vi "frontPanel.vi"() -> ()   [LabVIEW 2020]
uses:
  C:/Users/DESKTOP-TLO0G68A/Desktop/instrumentationLV/Thorlabs.MotionControl.Controls.dll
  Thorlabs.MotionControl.Controls.dll
  C:/Users/DESKTOP-TLO0G68A/Desktop/instrumentationLV/ThorLabs.MotionControl.KCube.DCServoCLI.dll
  ThorLabs.MotionControl.KCube.DCServoCLI.dll
panel:
  in  "KCubeDCServoControl 1":refnum<k24>(container)
  in  "?":bool
  in  "?":bool
  in  "?":bool
  in  "Direction 2":i32(ring)=1 items=["Forward"=1, "Backward"=2]
  in  "Step Size 2":dbl
  in  "KCubeDCServoControl 2":refnum<k24>(container)
  in  "?":bool
  in  "?":bool
  in  "?":bool
  in  "Direction":i32(ring)=1 items=["Forward"=1, "Backward"=2]
  in  "Step Size":dbl
  in  "x steps":dbl
  in  "NPLC":dbl
  in  "# of pts":dbl
  in  "velocity":dbl
  in  "ending voltage":dbl
  in  "starting voltage":dbl
  in  "Oscilloscope VISA addr":refnum<visa-resource-name>
  in  "Keithley VISA addr":refnum<visa-resource-name>
  in  "acceleration":dbl
  in  "step size":dbl=0.025
  in  "y steps":dbl
  in  "Starting y":dbl
  in  "Starting x":dbl
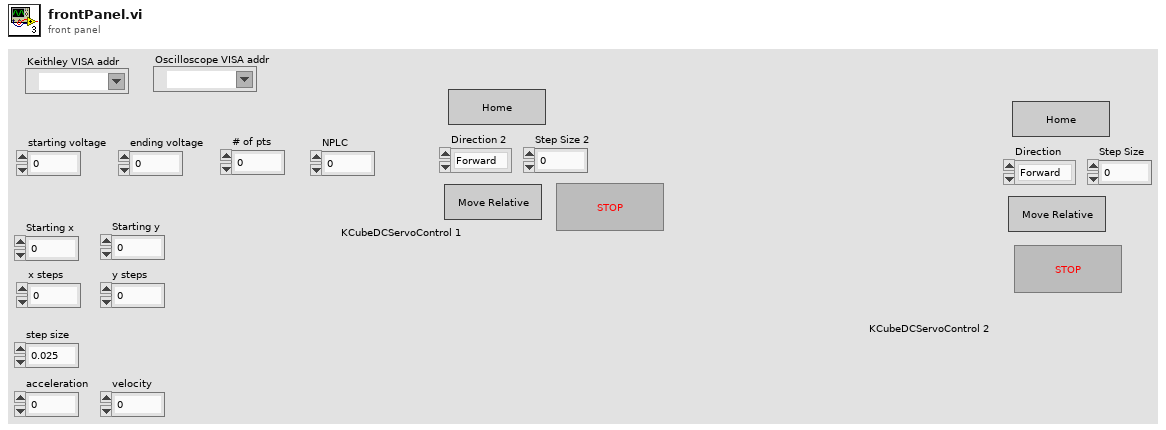
[diagram p1: front panel]
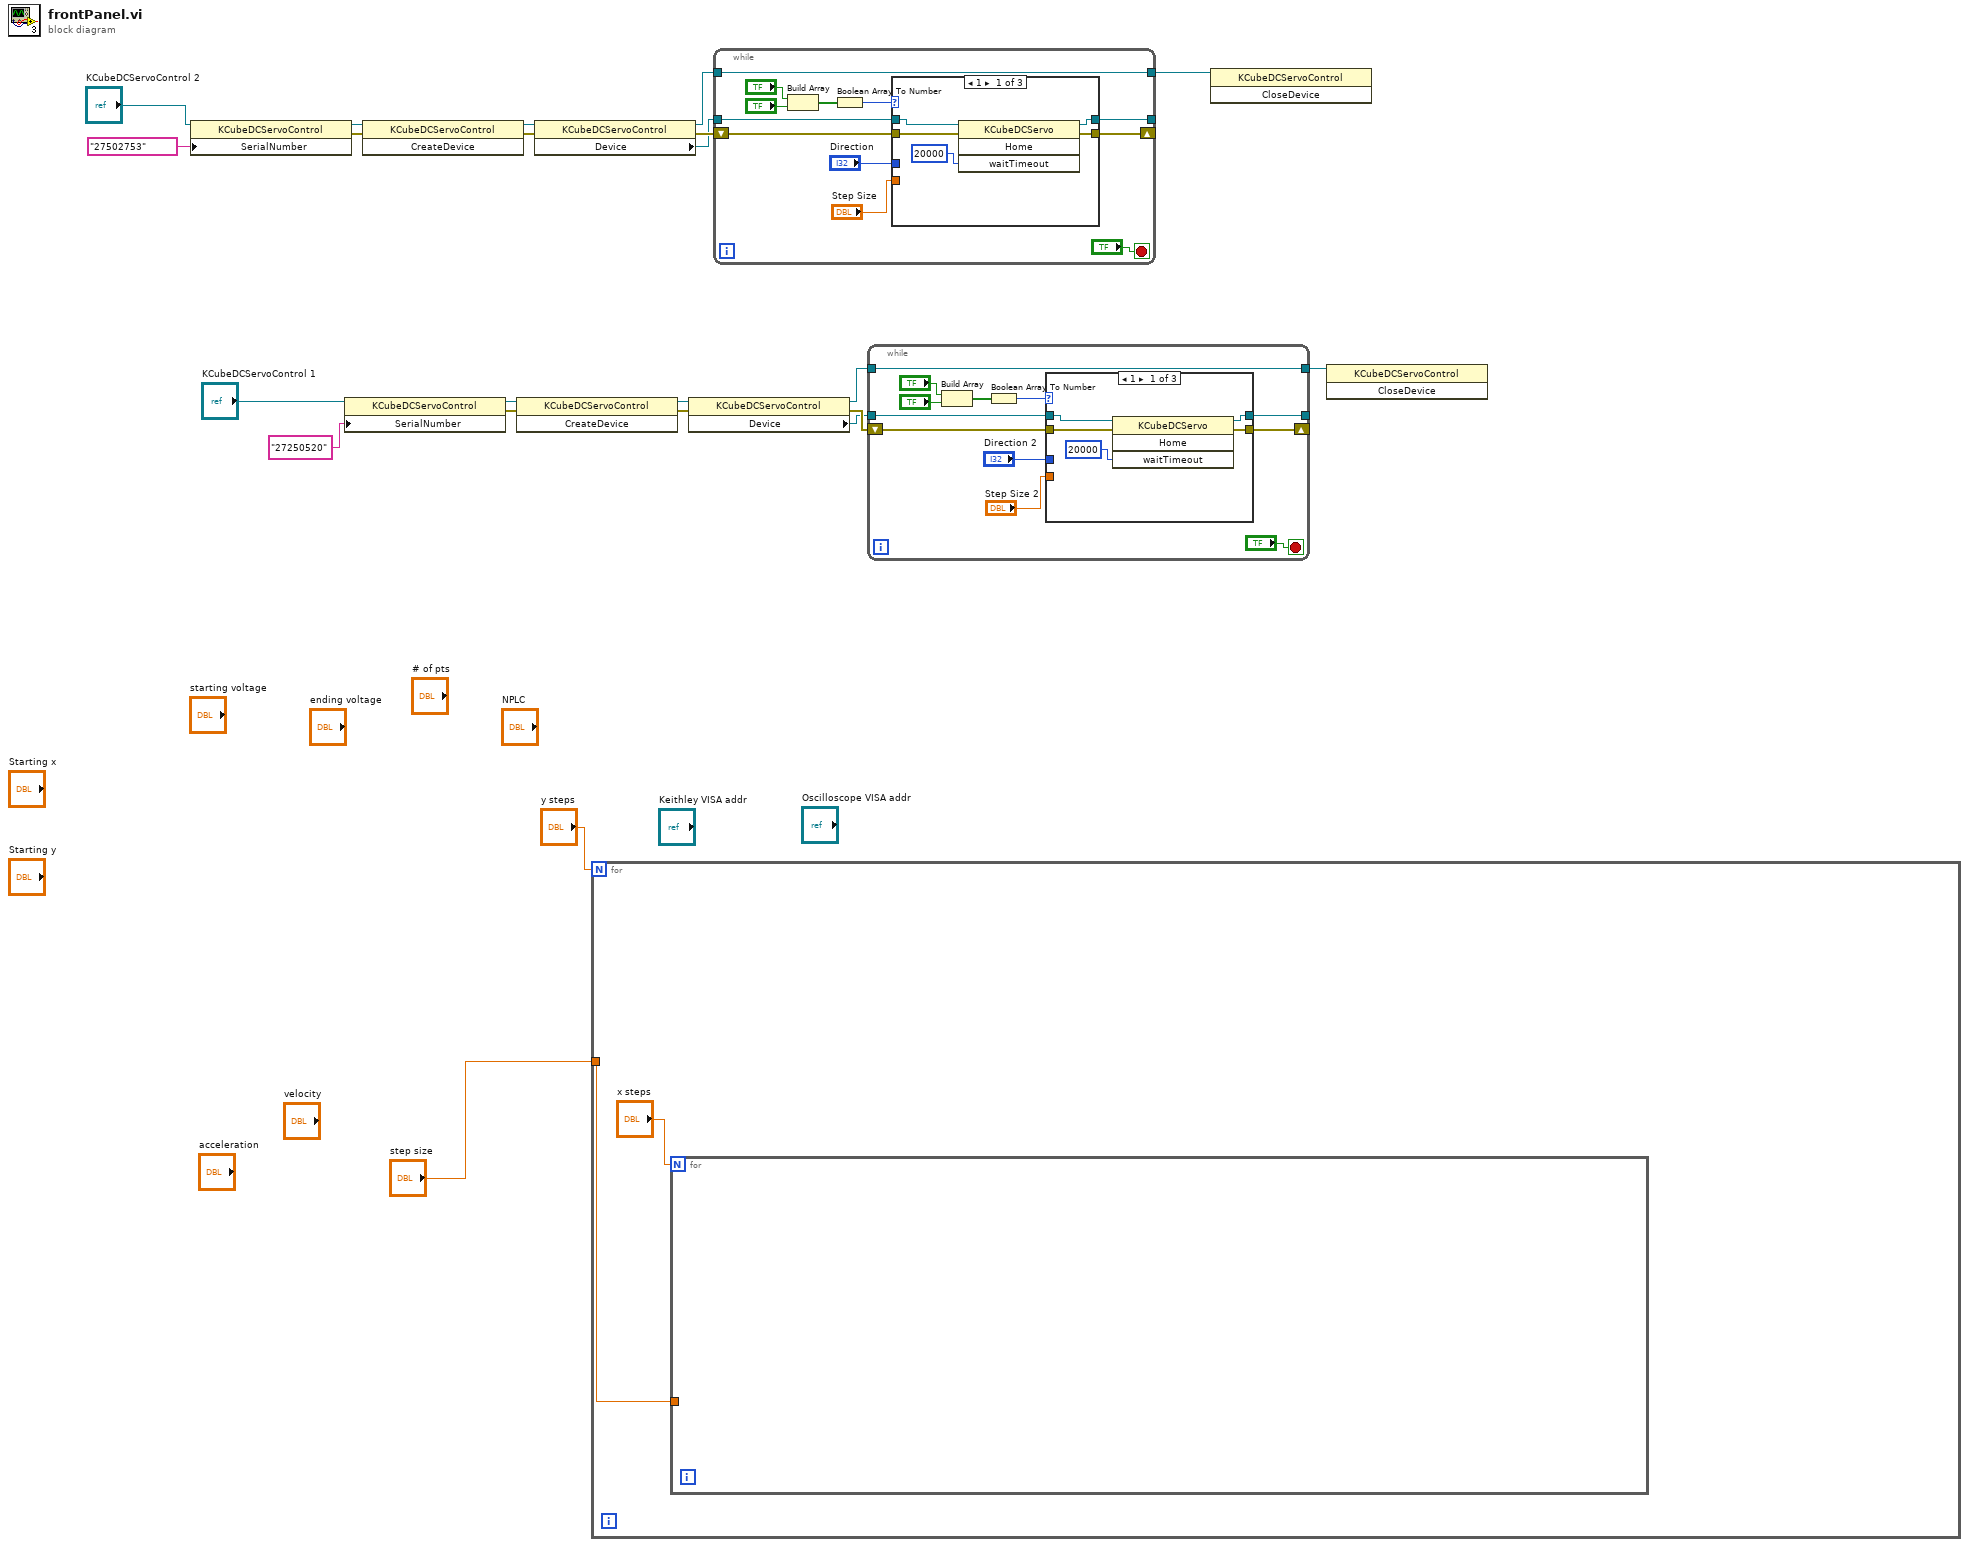
[diagram p0: block diagram]
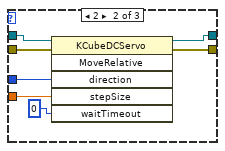
[diagram p2: hidden frame]
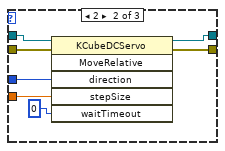
[diagram p4: hidden frame]
diagram:
  n1 = property class="KCubeDCServoControl"(reference="KCubeDCServoControl 2", "SerialNumber"="27502753") -> (reference out=w18:refnum<k24>, error out=w16:errorcluster)  [unwired: 1 in]
  n2 = property class="KCubeDCServoControl"(reference="KCubeDCServoControl 1", "SerialNumber"="27250520") -> (reference out=w8:refnum<k24>, error out=w6:errorcluster)  [unwired: 1 in]
  n3 = invoke class="KCubeDCServoControl" method="CreateDevice"(reference=w18, error in=w16) -> (reference out=w17:refnum<k24>, error out=w15:errorcluster)  [unwired: 1 in, 1 out]
  n4 = invoke class="KCubeDCServoControl" method="CreateDevice"(reference=w8, error in=w6) -> (reference out=w7:refnum<k24>, error out=w5:errorcluster)  [unwired: 1 in, 1 out]
  n5 = property class="KCubeDCServoControl"(reference=w17, error in=w15) -> (reference out=w14:refnum<k24>, error out=w13:errorcluster, "Device"=w12:refnum<k24>)
  n6 = for {
    N: "y steps" -> [_]
    tunnel: "step size" -> [w23]
    n7 = for {
      N: "x steps" -> [_]
      tunnel: w23 -> [_]
    }
  }
  n8 = property class="KCubeDCServoControl"(reference=w7, error in=w5) -> (reference out=w4:refnum<k24>, error out=w3:errorcluster, "Device"=w2:refnum<k24>)
  n9 = while {
    tunnel: [w29] -> _
    shift-right: [w31] -> _
    shift-left: w13 -> [w30]
    tunnel: w12 -> [w28]
    tunnel: [w25] -> w20
    tunnel: w14 -> [w25]
    stop <- "?" stop-if-true
    n10 = Build Array("?", "?") -> (w33:bool[])
    n11 = Boolean Array To Number(Boolean array=w33) -> (number=w32:u32)
    n12 = case shown="1" w32 {
      tunnel: w28 -> [w41 w48 w49]
      tunnel: [w37 w42 w50] -> w31
      tunnel: w30 -> [w38 w43 w50]
      tunnel: [w39 w47 w49] -> w29
      tunnel: "Direction" -> [_ w46 _]
      tunnel: "Step Size" -> [_ w45 _]
      frame 1 {
        n13 = invoke class="KCubeDCServo" method="Home"(reference=w41, error in=w38, "waitTimeout"=20000) -> (reference out=w39:refnum<k24>, error out=w37:errorcluster)  [unwired: 1 in, 2 out]
      }
      frame 2 {
        n14 = invoke class="KCubeDCServo" method="MoveRelative"(reference=w48, error in=w43, "direction"=w46, "stepSize"=w45, "waitTimeout"=0) -> (reference out=w47:refnum<k24>, error out=w42:errorcluster)  [unwired: 1 in, 4 out]
      }
      frame Default {
      }
    }
  }
  n15 = while {
    tunnel: [w55] -> _
    shift-right: [w57] -> _
    shift-left: w3 -> [w56]
    tunnel: w2 -> [w54]
    tunnel: [w51] -> w10
    tunnel: w4 -> [w51]
    stop <- "?" stop-if-true
    n16 = Build Array("?", "?") -> (w59:bool[])
    n17 = Boolean Array To Number(Boolean array=w59) -> (number=w58:u32)
    n18 = case shown="1" w58 {
      tunnel: w54 -> [w67 w74 w75]
      tunnel: [w63 w68 w76] -> w57
      tunnel: w56 -> [w64 w69 w76]
      tunnel: [w65 w73 w75] -> w55
      tunnel: "Direction 2" -> [_ w72 _]
      tunnel: "Step Size 2" -> [_ w71 _]
      frame 1 {
        n19 = invoke class="KCubeDCServo" method="Home"(reference=w67, error in=w64, "waitTimeout"=20000) -> (reference out=w65:refnum<k24>, error out=w63:errorcluster)  [unwired: 1 in, 2 out]
      }
      frame 2 {
        n20 = invoke class="KCubeDCServo" method="MoveRelative"(reference=w74, error in=w69, "direction"=w72, "stepSize"=w71, "waitTimeout"=0) -> (reference out=w73:refnum<k24>, error out=w68:errorcluster)  [unwired: 1 in, 4 out]
      }
      frame Default {
      }
    }
  }
  n21 = invoke class="KCubeDCServoControl" method="CloseDevice"(reference=w20) -> ()  [unwired: 2 in, 3 out]
  n22 = invoke class="KCubeDCServoControl" method="CloseDevice"(reference=w10) -> ()  [unwired: 2 in, 3 out]
